vi "HP4192A_1.vi"(2 "save to:":path) -> (3 "Z":cluster{dbl[], dbl[]}(graph), 4 "R":cluster{dbl[], dbl[]}(graph), 5 "phase angle":cluster{dbl[], dbl[]}(graph), 6 "X":cluster{dbl[], dbl[]}(graph))   [LabVIEW 2012]
doc: "HP 4192A LF IMPEDANCE ANALYZER\n\nDEFAULTS: GPIB addr: 17\n Function A: Z/Y\n Function B: DEG\n Frequency: 100 Khz\n Circuit Mode: AUTO\n Trigger: INTERNAL\n Osc. Level: 1.0V\n DC Bias: OFF\n Bias Level: 0V\n\n\nGPIB PROGRAMMING NOTES: The command format consists of an ASCII string of control codes and numeric parameters. Commas act as seperators between individual commands. Whenever a numeric parameter is used, it is followed by 'EN,' signifying 'ENTER'. The 4192A is set to output an SRQ when a measurment is completed. The GPIB address is briefly shown in the 'DISPLAY A' window when the 4192A is first turned on. During remote operation, the 4192A front panel Remote LED will be activated verifying communication has been established. Consult the operation Manual Section 3, p68 for further description of the GPIB and control codes.\n\nINTERACTIVE OPERATION: The 4192A Virtural Instrument (VI) provides impedance measurments of circuits or components under test. 'FUNCTION A' selects the following measurments: Capacitance, Inductance, Resistance / Conductance, and Impedance / Addmittance. 'FUNCTION B' selects a characteristic of the measurment which includes: quality factor (Q), dissipation factor (D), resistance, or conductance. These parameters apply to L & C measurments. 'FUNCTION B' can also select Radians and Degrees which apply to Z/Y measurments. 'TEST SIGNAL FREQUENCY' has a range of 5Hz to 13Mhz. 'OSC LEVEL' has a range of 5mV to 1.1V. 'CIRCUIT MODE' selects between Auto mode, series circuits, and parallel circuits. The Series Mode applies to Z, R, and X measurments and the Parallel Mode applies to Y, G, and B measurments. The 'TRIGGER' control selects between Hold/Manual, External, and Internal Triggering. To operate the instrument interactively, select the desired options on the VI front panel and execute. The measurment results will be displayed in the 'DISPLAY A' and 'DISPLAY B' windows when execution is complete. Additionally, the 4192A can make bias or frequency sweep measurments using the '4192A Sweep' VI once the 4192A VI has been set up. The '4192A Sweep' provides bias and sweep options, start up and start down options, and selection between log or linear sweep.\n\nPROGRAMMATIC OPERATION: A example program is included in this package showing the 4192A and 4192A Sweep used programmatically. The following values can be used as inputs to the 4192A ICON; the ICON and connector pane are shown below:\n\n \n\n\nFREQUENCY: 5 to 13E6 Hz\n \nOSC. LEVEL: 5E-3 to 1.1V\n\nFUNCTION A INPUT: 0=Z/Y\n 1=R/G\n 2=L\n 3=C\n\nFUNCTION B INPUT: 0=DEG/Q\n 1=RAD/Q\n 2=R/G\n\nCIRCUIT MODE INPUT: 0=AUTO\n 1=SERIES\n 2=PARALLEL\n\nTRIGGER INPUT: 0=HOLD/MANUAL\n 1=EXTERNAL\n 2=INTERNAL\n\nBIAS: Binary Switch\n\nBIAS (V): -35 to 35V"
uses:
  <vilib>/Utility/file.llb/Write To Spreadsheet File (DBL).vi
panel:
  in  "log sweep":i16(slide)=1 scale=0.0..1.0 scale format="%.2f"
  in  "GPIB address":string="17"
  out "capacitance\nvalue (F)":dbl format="%.3e"
  in  "step freq (Hz)":dbl=82644.0 min=5.0 max=13000000.0 format="%.3e"
  in  "stop freq (Hz)":dbl=10000000.0 min=5.0 max=13000000.0 format="%.3e"
  in  "start freq (Hz)":dbl=10.0 min=5.0 max=13000000.0 format="%.3e"
  # "© Copyright 1993 National Instruments Corporation.  All Rights Reserved."
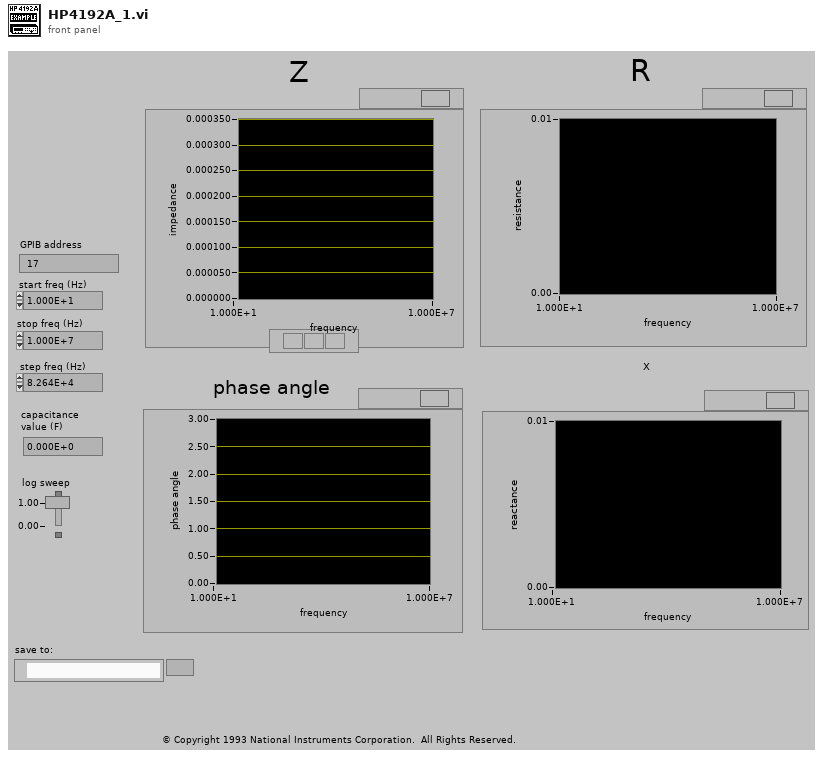
[diagram p1: front panel]
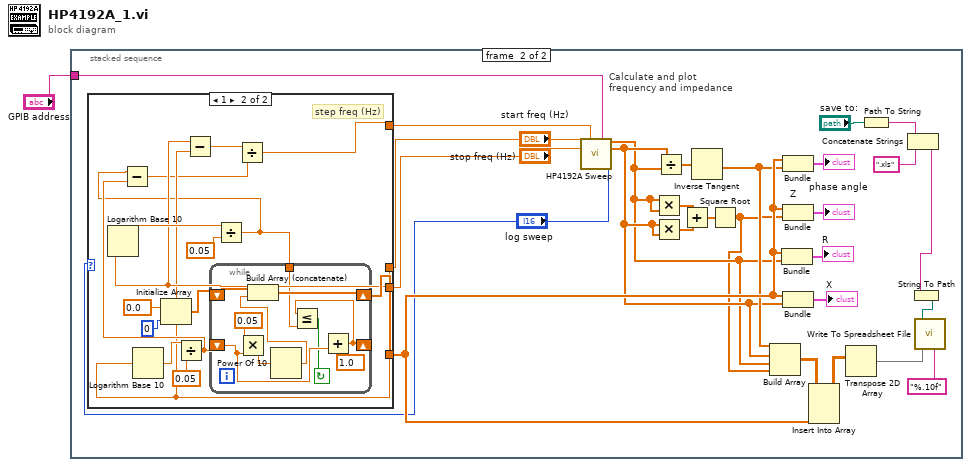
[diagram p0: block diagram]
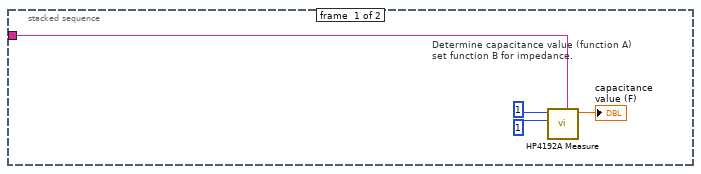
[diagram p2: hidden frame]
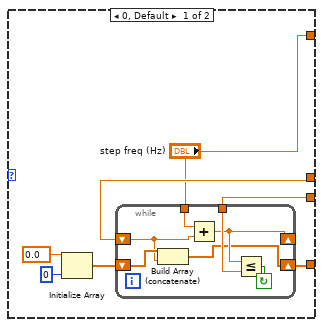
[diagram p3: hidden frame]
diagram:
  n1 = stacked-sequence {
    tunnel: "GPIB address" -> [w2 w32]
    frame #0 {
      # "Determine capacitance value (function A)\nset function B for impedance."
      n2 = call "HP4192A Measure.vi"("GPIB addess"=w2, "function B (deg q:0)"=1, "function A (z/y:0)"=1) -> ("display A"=→"capacitance\nvalue (F)":dbl)  [unwired: 7 in, 1 out]
    }
    frame #1 {
      # "Calculate and plot\nfrequency and impedance"
      n3 = case shown="1" "log sweep" {
        tunnel: "stop freq (Hz)" -> [w39 w52]
        tunnel: "start freq (Hz)" -> [w35 w51]
        tunnel: [w34 w54] -> w27
        tunnel: ["step freq (Hz)" w49] -> w20
        frame 0, Default {
          n4 = Initialize Array(0.0 ("element"), 0 ("dimension size")) -> (w36:dbl[])
          n5 = while {
            shift-right: [w43] -> _
            shift-left: w35 -> [w41]
            tunnel: "step freq (Hz)" -> [w46]
            tunnel: w39 -> [w45]
            shift-right: [w40] -> w34
            shift-left: w36 -> [w42]
            stop <- w44 continue-if-true
            n6 = Build Array (concatenate)(w42, w41) -> (w40:dbl[])
            n7 = Add(x=w46, y=w41) -> (x+y=w43:dbl)
            n8 = Less Or Equal?(x=w43, y=w45) -> (x <= y?=w44:bool)
          }
        }
        frame 1 {
          # "step freq (Hz)"
          n9 = Logarithm Base 10(1:w52) -> (0:w55:dbl)
          n10 = Logarithm Base 10(1:w51) -> (0:w58:dbl)
          n11 = Initialize Array(0.0 ("element"), 0 ("dimension size")) -> (w59:dbl[])
          n12 = Divide(x=w58, y=0.05) -> (x/y=w53:dbl)
          n13 = Subtract(x=w52, y=w51) -> (x-y=w50:dbl)
          n14 = Divide(x=w55, y=0.05) -> (x/y=w48:dbl)
          n15 = Subtract(x=w48, y=w53) -> (x-y=w47:dbl)
          n16 = while {
            shift-right: [w69] -> w54
            shift-left: w59 -> [w71]
            shift-right: [w62] -> _
            shift-left: w53 -> [w65]
            tunnel: w48 -> [w63]
            stop <- w64 continue-if-true
            n17 = Multiply(x=0.05, y=w65) -> (x*y=w68:dbl)
            n18 = Power Of 10(x=w68) -> (10^x=w67:dbl)
            n19 = Build Array (concatenate)(w71, w67) -> (w69:dbl[])
            n20 = Add(x=1.0, y=w65) -> (x+y=w62:dbl)
            n21 = Less Or Equal?(x=w62, y=w63) -> (x <= y?=w64:bool)
          }
          n22 = Divide(x=w50, y=w47) -> (x/y=w49:dbl)
        }
      }
      n23 = call "HP4192A Sweep.vi"("start freq (Hz)"="start freq (Hz)", "step freq (Hz)"=w20, "GPIB address"=w32, "stop freq (Hz)"="stop freq (Hz)", "log sweep"="log sweep") -> ("display A"=w8:dbl[], "display B"=w9:dbl[])  [unwired: 6 in, 3 out]
      n24 = Multiply(x=w8, y=w8) -> (x*y=w12:dbl[])
      n25 = Multiply(x=w9, y=w9) -> (x*y=w11:dbl[])
      n26 = Divide(x=w9, y=w8) -> (x/y=w14:dbl[])
      n27 = Add(x=w12, y=w11) -> (x+y=w13:dbl[])
      n28 = Inverse Tangent(1:w14) -> (0:w10:dbl[])
      n29 = Square Root(x=w13) -> (sqrt(x)=w7:dbl[])
      n30 = Build Array(w10, w9, w8, w7) -> (w30:dbl[][])
      n31 = Bundle(w27, "display A"=w8) -> (→"R":cluster{dbl[], "display A":dbl[]})  [unwired: 1 in]
      n32 = Bundle(w27, w10) -> (→"phase angle":cluster{dbl[], dbl[]})  [unwired: 1 in]
      n33 = Bundle(w27, w7) -> (→"Z":cluster{dbl[], dbl[]})  [unwired: 1 in]
      n34 = Bundle(w27, "display B"=w9) -> (→"X":cluster{dbl[], "display B":dbl[]})  [unwired: 1 in]
      n35 = Insert Into Array(array=w30, new element=w27) -> (w29:dbl[][])  [unwired: 2 in]
      n36 = Transpose 2D Array(2D array=w29) -> (transposed array=w31:dbl[][])
      n37 = Path To String(path="save to:") -> (string=w15:string)
      n38 = Concatenate Strings(w15, ".xls") -> (w22:string)
      n39 = String To Path(string=w22) -> (path=w23:path)
      n40 = call-poly <vilib>:"Write To Spreadsheet File.vi"("format (%.3f)"="%.10f", "2D data"=w31, "file path (dialog if empty)"=w23) -> ()  [unwired: 5 in, 1 out]
    }
  }
